vi "GetPosition.vi"(8 "error in (no error)":errorcluster, 10 "Setup":T1={"Scaling (pixels/mm)"=1.0, "Tool Diameter (inch)"=0.25, "Origin location"={"x (mm)"=10, "y (mm)"=300}, "Wood dim"={"width (inch)"=10.0, "height (inch)"=300.0}}, 11 "VISA Refnum in":refnum<visa-resource-name>) -> (0 "error out":errorcluster, 1 "success?":bool, 2 "new picture":picture, 3 "Position":T2)   [LabVIEW 2024]
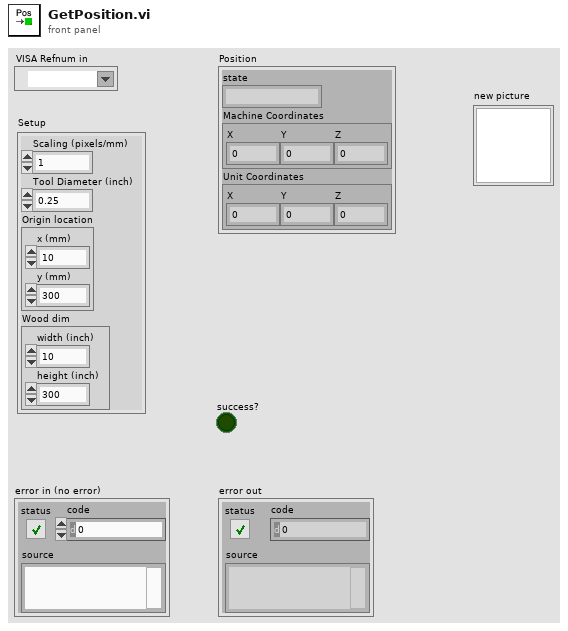
[diagram p1: front panel]
types:
  T1 = cluster{"Scaling (pixels/mm)":dbl, "Tool Diameter (inch)":dbl, "Origin location":cluster{"x (mm)":i16, "y (mm)":i16}, "Wood dim":cluster{"width (inch)":dbl, "height (inch)":dbl}}
  T2 = cluster{"state":string, "Machine Coordinates":cluster{"X":dbl, "Y":dbl, "Z":dbl}, "Unit Coordinates":cluster{"X":dbl, "Y":dbl, "Z":dbl}}
  T3 = cluster{"String out":string, cluster{dbl, dbl, dbl}, cluster{dbl, dbl, dbl}}
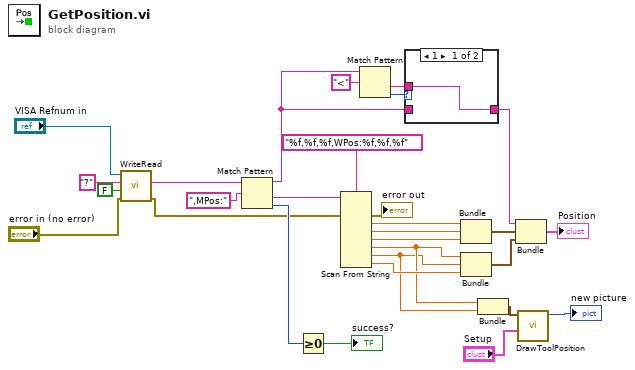
[diagram p0: block diagram]
diagram:
  n1 = call "WriteRead.vi"("error in (no error)"="error in (no error)", "warn?"=FALSE, "String in"="?" ("string"), "VISA Refnum in"="VISA Refnum in") -> ("error out"=w13:errorcluster, "String out"=w16:string)  [unwired: 4 in, 2 out]
  n2 = Match Pattern(string=w16, regular expression=",MPos:") -> (before substring=w6:string, after substring=w14:string, offset past match=w20:i32)  [unwired: 1 in, 1 out]
  n3 = Greater Or Equal To 0?(x=w20) -> (x >= 0?=→"success?":bool)
  n4 = Scan From String(format string="%f,%f,%f,WPos:%f,%f,%f", input string=w14, error in=w13) -> (error out=→"error out":errorcluster, output 1=w24:dbl, output 2=w25:dbl, output 3=w26:dbl, output 4=w3:dbl, output 5=w2:dbl, output 6=w27:dbl)  [unwired: 7 in, 2 out]
  n5 = Match Pattern(string=w6, regular expression="<") -> (after substring=w5:string, offset past match=w8:i32)  [unwired: 1 in, 2 out]
  n6 = case shown="1" w8 {
    tunnel: [w30 w31] -> w7
    tunnel: w6 -> [_ w31]
    tunnel: w5 -> [w30 _]
    frame 1 {
    }
    frame Default {
    }
  }
  n7 = Bundle(w24, w25, w26) -> (w23:cluster{dbl, dbl, dbl})  [unwired: 1 in]
  n8 = Bundle(w3, w2, w27) -> (w22:cluster{dbl, dbl, dbl})  [unwired: 1 in]
  n9 = Bundle(w3, w2) -> (w1:cluster{dbl, dbl})  [unwired: 1 in]
  n10 = Bundle("String out"=w7, w23, w22) -> (→"Position":T3)  [unwired: 1 in]
  n11 = call "DrawToolPosition.vi"("Setup"="Setup", "dot position"=w1) -> ("blob"=→"new picture":picture)  [unwired: 9 in]
